vi "Display QDList Info In QuickBox.vi"(8 "error in (no error)":errorcluster, 9 "QDFunction Acronym(\"\")":string, 10 "QDFunction Name(\"\")":string, 11 "NormalQDFunc in":refnum<class "QDList.lvclass">) -> (0 "error out":errorcluster, 2 "Content For Display":string, 3 "NormalQDFunc out":refnum<class "QDList.lvclass">)   [LabVIEW 2015, in "QDList.lvclass"]
uses:
  QDList.lvclass
  QDList.lvclass/QDList.ctl
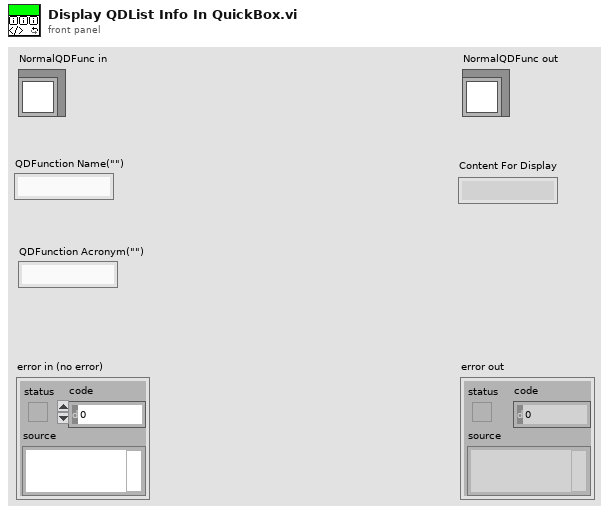
[diagram p1: front panel]
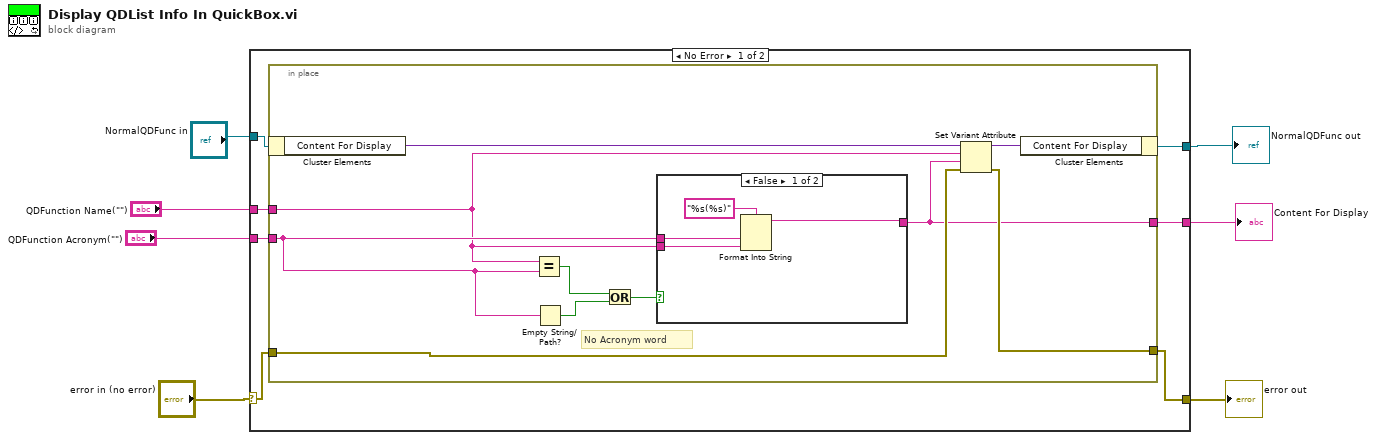
[diagram p0: block diagram]
diagram:
  n1 = case shown="No Error" "error in (no error)" {
    selector: "error in (no error)" -> [w9 w31]
    tunnel: [w14 _] -> w7
    tunnel: "NormalQDFunc in" -> [w13 w30]
    tunnel: [w8 w31] -> w4
    tunnel: [w12 w30] -> w3
    tunnel: "QDFunction Name(\"\")" -> [w11 _]
    tunnel: "QDFunction Acronym(\"\")" -> [w10 _]
    frame No Error {
      n2 = in-place {
        in-place-border: [w15] -> w14
        in-place-border: w11 -> [w18]
        in-place-border: w10 -> [w21]
        in-place-border: w9 -> [w17]
        in-place-border: [w16] -> w8
        # "No Acronym word"
        n3 = in-place-cluster #1(w13) -> ("Content For Display"=w20:variant)
        n4 = Equal?(x=w18, y=w21) -> (x = y?=w24:bool)
        n5 = Empty String/Path?(string/path=w21) -> (empty?=w23:bool)
        n6 = Or(x=w24, y=w23) -> (x .or. y?=w22:bool)
        n7 = case shown="False" w22 {
          tunnel: [w27 w29] -> w15
          tunnel: w21 -> [w26 _]
          tunnel: w18 -> [w25 w29]
          frame False {
            n8 = Format Into String(format string="%s(%s)", w26, w25) -> (resulting string=w27:string)  [unwired: 2 in, 1 out]
          }
          frame True {
          }
        }
        n9 = Set Variant Attribute(Variant=w20, name=w18, value=w15, error in=w17) -> (Variant out=w19:variant, error out=w16:errorcluster)  [unwired: 1 out]
        n10 = in-place-cluster #1("Content For Display"=w19) -> (w12:refnum<class "QDList.lvclass">)
      }
    }
    frame Error {
    }
  }
  "error out" <- w4
  "NormalQDFunc out" <- w3
  "Content For Display" <- w7
